vi "VISA.ID Query.vi"(6 "Timeout":u32=2000, 8 "error in":errorcluster, 10 "write data":string="*IDN?", 11 "VISA resource name":refnum<visa-resource-name>) -> (0 "error out":errorcluster, 2 "read data":string)   [LabVIEW 2018]
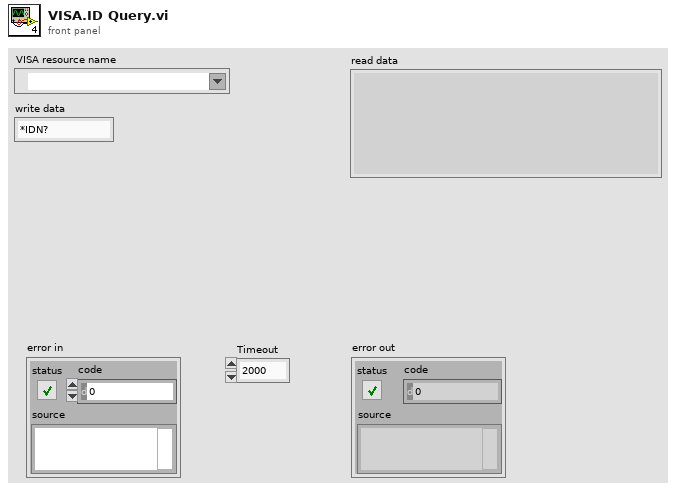
[diagram p1: front panel]
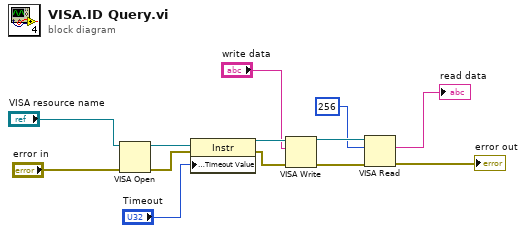
[diagram p0: block diagram]
diagram:
  n1 = VISA Open(error in (no error)="error in", VISA resource name="VISA resource name") -> (VISA resource name=w1:refnum<visa-resource-name>, error out=w4:errorcluster)  [unwired: 3 in]
  n2 = property class="Instr"(reference=w1, error in=w4, "General Settings:Timeout Value"="Timeout") -> (reference out=w10:refnum<visa-resource-name>, error out=w9:errorcluster)
  n3 = VISA Write(VISA resource name=w10, write buffer="write data", error in (no error)=w9) -> (VISA resource name out=w13:refnum<visa-resource-name>, error out=w8:errorcluster)  [unwired: 1 out]
  n4 = VISA Read(VISA resource name=w13, byte count=u32 256, error in (no error)=w8) -> (read buffer=→"read data":string, error out=→"error out":errorcluster)  [unwired: 2 out]
